vi "rs3 create sensor.vi"(8 "error in (no error)":errorcluster, 10 "Sensor index":i32, 11 "Sensor list":u64) -> (0 "error out":errorcluster, 1 "Sensor out":u64, 2 "error":u64, 3 "Sensor list out":u64)   [LabVIEW 2023]
doc: "Creates a SENSOR based on an input index to a SENSOR LIST.\n\nINPUT: \nSensor list Array of sensor handles\nIndex Input index \n\nOUTPUT:\nSensor out The SENSOR handle to be used for all subsequent communication\nError 0=no error"
panel:
  # "RS3 Create Sensor"
  # "(C) 2017 Intel Corp.,  AGJ"
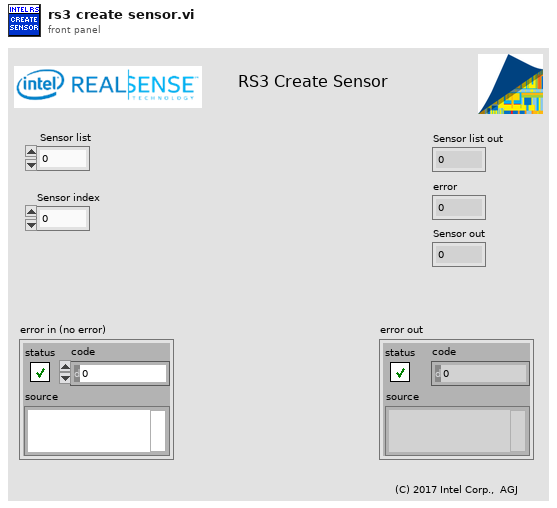
[diagram p1: front panel]
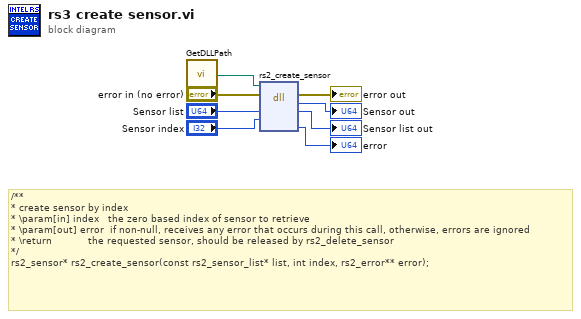
[diagram p0: block diagram]
diagram:
  # "/**\n* create sensor by index\n* \\param[in] index   the zero based index of sensor to retrieve\n* \\param[out] error  if non-null, receives any error that occurs during this call, otherwise, errors are ignored\n* \\return            the requested sensor, should be released by rs2_delete_sensor\n*/\nrs2_sensor* rs2_create_sensor(const rs2_sensor_list* list, int index, rs2_error** error);"
  n1 = call "GetDLLPath.vi"() -> ("DLL Path"=w1:path)
  n2 = dll-call lib="C:/STEAMSyndicate/RealSenseWrappers/VI Wrappers (add ons) Public/RealSense/realsense2.dll" fn="rs2_create_sensor"(path in=w1, error in="error in (no error)", "sensor list"="Sensor list", "index"="Sensor index") -> (error out=→"error out":errorcluster, "sensor"=→"Sensor out":u64, "sensor list"=→"Sensor list out":u64, "error"=→"error":u64)  [unwired: 3 in, 1 out]
